vi "Page_Info_Read.vi"(6 "ctlReferences":T1, 8 "error in (no error)":errorcluster, 11 "AB_InteropAssembly in":refnum<class "AB_InteropAssembly.lvclass">) -> (0 "error out":errorcluster, 3 "AB_InteropAssembly out":refnum<class "AB_InteropAssembly.lvclass">)   [LabVIEW 2020, in "AB_InteropAssembly.lvclass"]
uses:
  <vilib>/AppBuilder/AB_Classes/InteropAssembly/AB_InteropAssembly.lvclass
  e:/builds/penguin/labview/branches/2020/dev/dist/vi.lib/AppBuilder/AB_Classes/Build/AB_Build.lvclass
  <resource>/Framework/Providers/Builds/AppBuilder/AB_UI_Page_Info_References.ctl
  <vilib>/AppBuilder/AB_Classes/InteropAssembly/AB_InteropAssembly.lvclass/AB_InteropAssembly.ctl
  <resource>/Framework/Providers/Common/provcom_StringGlobals.vi
  <vilib>/AppBuilder/AB_Classes/Application/AB_Application.lvclass
  <vilib>/AppBuilder/AB_Classes/Build/AB_Build.lvclass
  <vilib>/AppBuilder/AB_Classes/Destination/AB_Destination.lvclass
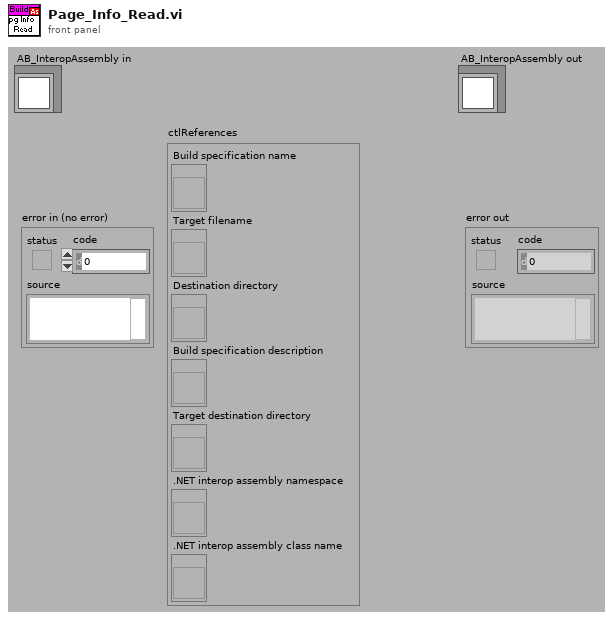
[diagram p1: front panel]
types:
  T1 = typedef "AB_UI_Page_Info_References.ctl" = cluster{"Build specification name":refnum<vi>, "Target filename":refnum<vi>, "Destination directory":refnum<vi>, "Build specification description":refnum<vi>, "Target destination directory":refnum<vi>, ".NET interop assembly namespace":refnum<vi>, ".NET interop assembly class name":refnum<vi>}
  T2 = typedef "AB_Build.ctl" = cluster{"buildSpecName":string, "buildSpecDescription":string, "destinations":refnum<class "AB_Destination.lvclass">[], "exclusionOption":T3, "defaultLanguage":string, "supportedLanguages":string[], "excludedDirectories":path[], "buildContext":refnum<vi>, "buildObject":T4, "preview":bool, "programatic":bool, "progressBarEvents":T5, "userLog_Path":path, "preActionID":string, "preAction_Path":path, "postActionID":string, "postAction_Path":path, "eng_checkForBrokenVIs?":bool, "eng_verboseLinkerErrors?":bool, "localDest_Path":path, "targetDest_Path":path, "removeVIObject":u16, "cache":refnum<class "PreviewCache.lvclass">, "use cache":bool, "previewCache_ID":string, "buildCache_ID":string, "eng_TempLocalDest_Path":path, "eng_collectDependencies?":bool, "versionInfo":cluster{"buildVersion":cluster{"major":u16, "minor":u16, "patch":u16, "build":u16}, "autoIncrement":bool}, "eng_enableVIChecksums":bool}
  T3 = typedef "AB_Exclusion_Option.ctl" = cluster{"typedefs":bool, "polymorphicVIs":bool, "unusedLibraryItems":bool, "modifyLibraryFile":bool, "edit-timeDependencies":bool, "inlineVIs":bool, "dependent PPLs":bool, "dependent DLLs":bool}
  T4 = typedef "ItemRef.ctl" = u64
  T5 = typedef "provcom_ProgressBar_Events.ctl" = cluster{"newJob":refnum<user-event>, "newItem":refnum<user-event>, "errorMsg":T6, "cancel":refnum<user-event>}
  T6 = typedef "mxLvBuildError.ctl" = refnum<user-event>
  T7 = typedef "AB_Destination.ctl" = cluster{"destName":string, "path":path, "libraryName":string, "preserveHierarchy":bool, "eng_inBuild":bool, "eng_libraryReference":refnum<vi>, "eng_restictAddToNewLibrary":bool}
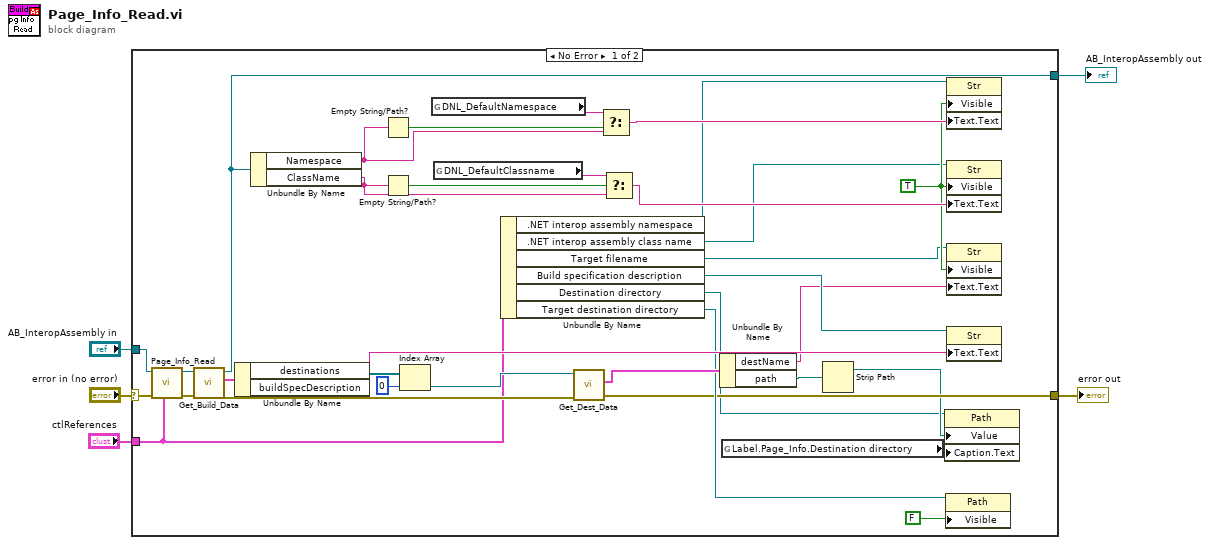
[diagram p0: block diagram]
diagram:
  n1 = case shown="No Error" "error in (no error)" {
    selector: "error in (no error)" -> [w23 w40]
    tunnel: "AB_InteropAssembly in" -> [w39 w41]
    tunnel: [w20 w40] -> w3
    tunnel: [w19 w41] -> w2
    tunnel: "ctlReferences" -> [w18 _]
    frame No Error {
      w13 = TRUE ("Visible")
      n2 = call-parent "Page_Info_Read.vi"("ctlReferences"=w18, "error in (no error)"=w23, "AB_Targetfile in"=w39) -> ("error out"=w22:errorcluster, "AB_Targetfile out"=w38:refnum<class "AB_InteropAssembly.lvclass">)  [unwired: 7 out]
      n3 = call <vilib>:"Get_Build_Data.vi"("error in (no error)"=w22, "Class in"=w38) -> ("error out"=w21:errorcluster, "data"=w37:T2, "Class out"=w19:refnum<class "AB_InteropAssembly.lvclass">)  [unwired: 7 out]
      n4 = Unbundle By Name(w37) -> ("destinations"=w36:refnum<class "AB_Destination.lvclass">[], "buildSpecDescription"=w32:string)
      n5 = Unbundle By Name(w19) -> ("Namespace"=w28:string, "ClassName"=w30:string)
      n6 = Empty String/Path?(string/path=w28) -> (empty?=w29:bool)
      n7 = Empty String/Path?(string/path=w30) -> (empty?=w31:bool)
      n8 = Index Array(array=w36, index=0) -> (element=w34:refnum<class "AB_Destination.lvclass">)
      n9 = global read "provcom_StringGlobals.vi" "DNL_DefaultNamespace"() -> (w15:string)
      n10 = global read "provcom_StringGlobals.vi" "DNL_DefaultClassname"() -> (w14:string)
      n11 = Unbundle By Name(w18) -> (".NET interop assembly namespace"=w12:refnum<vi>, ".NET interop assembly class name"=w11:refnum<vi>, "Target filename"=w9:refnum<vi>, "Build specification description"=w8:refnum<vi>, "Destination directory"=w10:refnum<vi>, "Target destination directory"=w24:refnum<vi>)
      n12 = call <vilib>:"Get_Dest_Data.vi"("error in (no error)"=w21, "Class in"=w34) -> ("error out"=w20:errorcluster, "destName"=w33:T7)  [unwired: 8 out]
      n13 = Select(t=w15, s=w29, f=w28) -> (s? t:f=w27:string)
      n14 = Select(t=w14, s=w31, f=w30) -> (s? t:f=w26:string)
      n15 = Unbundle By Name(w33) -> ("destName"=w7:string, "path"=w17:path)
      n16 = global read "provcom_StringGlobals.vi" "Label.Page_Info.Destination directory"() -> (w6:string)
      n17 = Strip Path(path=w17) -> (stripped path=w16:path)  [unwired: 1 out]
      n18 = property class="Path"(reference=w10, "Value"=w16, "Caption.Text"=w6) -> ()  [unwired: 1 in, 2 out]
      n19 = property class="Path"(reference=w24, "Visible"=FALSE) -> ()  [unwired: 1 in, 2 out]
      n20 = property class="Str"(reference=w12, "Visible"=w13, "Text.Text"=w27) -> ()  [unwired: 1 in, 2 out]
      n21 = property class="Str"(reference=w11, "Visible"=w13, "Text.Text"=w26) -> ()  [unwired: 1 in, 2 out]
      n22 = property class="Str"(reference=w9, "Visible"=w13, "Text.Text"=w7) -> ()  [unwired: 1 in, 2 out]
      n23 = property class="Str"(reference=w8, "Text.Text"=w32) -> ()  [unwired: 1 in, 2 out]
    }
    frame Error {
    }
  }
  "error out" <- w3
  "AB_InteropAssembly out" <- w2
